vi "arm.vi"() -> ()   [LabVIEW 2014]
panel:
  in  "Controller Daisy Chain Position (1 - 4)":u8=1
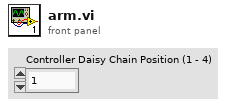
[diagram p1: front panel]
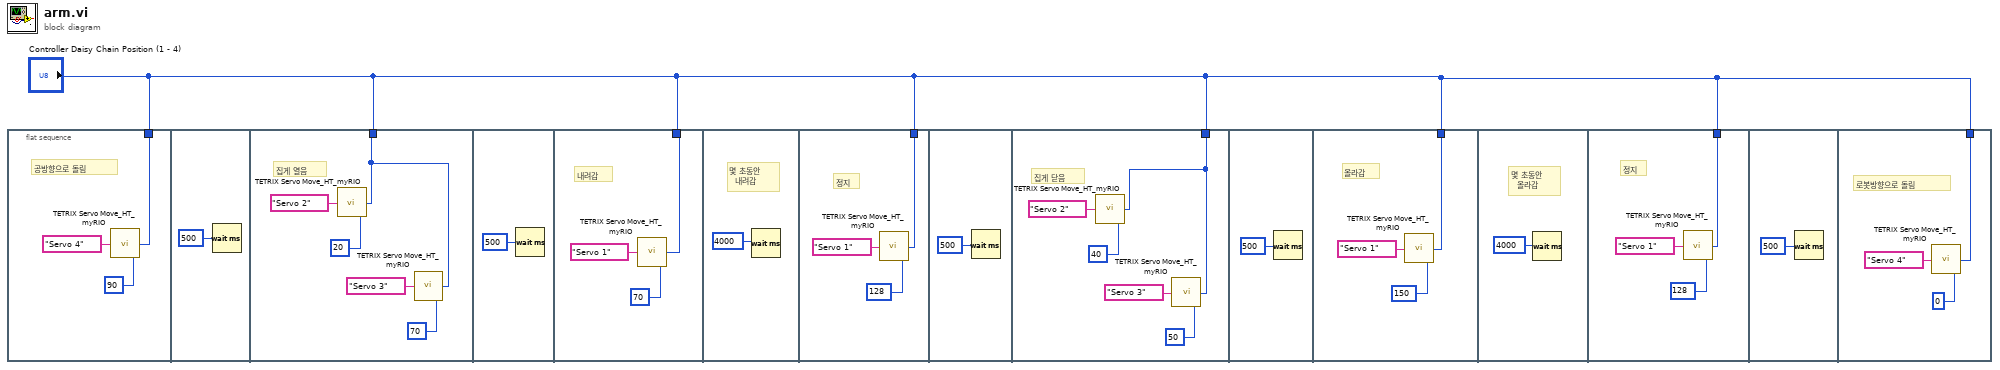
[diagram p0: block diagram]
diagram:
  n1 = flat-sequence {
    tunnel: "Controller Daisy Chain Position (1 - 4)" -> [w3]
    tunnel: "Controller Daisy Chain Position (1 - 4)" -> [w7]
    tunnel: "Controller Daisy Chain Position (1 - 4)" -> [w14]
    tunnel: "Controller Daisy Chain Position (1 - 4)" -> [w16]
    tunnel: "Controller Daisy Chain Position (1 - 4)" -> [w20]
    tunnel: "Controller Daisy Chain Position (1 - 4)" -> [w26]
    tunnel: "Controller Daisy Chain Position (1 - 4)" -> [w31]
    tunnel: "Controller Daisy Chain Position (1 - 4)" -> [w34]
    frame #0 {
      # "공방향으로 돌림"
      n2 = call <vilib>:"TETRIX Servo Move_HT_myRIO.vi"("Servo Position (0 - 255)"=u8 90, "Controller Daisy Chain Position (1 - 4)"=w3, "Select Servo"="Servo 4") -> ()  [unwired: 2 in, 1 out]
    }
    frame #1 {
      n3 = Wait (ms)(milliseconds to wait=u32 500 ("대기 시간(ms)")) -> ()  [unwired: 1 out]
    }
    frame #2 {
      # "집게 열음"
      n4 = call <vilib>:"TETRIX Servo Move_HT_myRIO.vi"("Servo Position (0 - 255)"=u8 20, "Controller Daisy Chain Position (1 - 4)"=w7, "Select Servo"="Servo 2") -> ()  [unwired: 2 in, 1 out]
      n5 = call <vilib>:"TETRIX Servo Move_HT_myRIO.vi"("Servo Position (0 - 255)"=u8 70, "Controller Daisy Chain Position (1 - 4)"=w7, "Select Servo"="Servo 3") -> ()  [unwired: 2 in, 1 out]
    }
    frame #3 {
      n6 = Wait (ms)(milliseconds to wait=u32 500 ("대기 시간(ms)")) -> ()  [unwired: 1 out]
    }
    frame #4 {
      # "내려감"
      n7 = call <vilib>:"TETRIX Servo Move_HT_myRIO.vi"("Servo Position (0 - 255)"=u8 70, "Controller Daisy Chain Position (1 - 4)"=w14, "Select Servo"="Servo 1") -> ()  [unwired: 2 in, 1 out]
    }
    frame #5 {
      # "몇 초동안\n  내려감"
      n8 = Wait (ms)(milliseconds to wait=u32 4000 ("대기 시간(ms)")) -> ()  [unwired: 1 out]
    }
    frame #6 {
      # "정지"
      n9 = call <vilib>:"TETRIX Servo Move_HT_myRIO.vi"("Servo Position (0 - 255)"=u8 128, "Controller Daisy Chain Position (1 - 4)"=w16, "Select Servo"="Servo 1") -> ()  [unwired: 2 in, 1 out]
    }
    frame #7 {
      n10 = Wait (ms)(milliseconds to wait=u32 500 ("대기 시간(ms)")) -> ()  [unwired: 1 out]
    }
    frame #8 {
      # "집게 닫음"
      n11 = call <vilib>:"TETRIX Servo Move_HT_myRIO.vi"("Servo Position (0 - 255)"=u8 40, "Controller Daisy Chain Position (1 - 4)"=w20, "Select Servo"="Servo 2") -> ()  [unwired: 2 in, 1 out]
      n12 = call <vilib>:"TETRIX Servo Move_HT_myRIO.vi"("Servo Position (0 - 255)"=u8 50, "Controller Daisy Chain Position (1 - 4)"=w20, "Select Servo"="Servo 3") -> ()  [unwired: 2 in, 1 out]
    }
    frame #9 {
      n13 = Wait (ms)(milliseconds to wait=u32 500 ("대기 시간(ms)")) -> ()  [unwired: 1 out]
    }
    frame #10 {
      # "올라감"
      n14 = call <vilib>:"TETRIX Servo Move_HT_myRIO.vi"("Servo Position (0 - 255)"=u8 150, "Controller Daisy Chain Position (1 - 4)"=w26, "Select Servo"="Servo 1") -> ()  [unwired: 2 in, 1 out]
    }
    frame #11 {
      # "몇 초동안\n  올라감"
      n15 = Wait (ms)(milliseconds to wait=u32 4000 ("대기 시간(ms)")) -> ()  [unwired: 1 out]
    }
    frame #12 {
      # "정지"
      n16 = call <vilib>:"TETRIX Servo Move_HT_myRIO.vi"("Servo Position (0 - 255)"=u8 128, "Controller Daisy Chain Position (1 - 4)"=w31, "Select Servo"="Servo 1") -> ()  [unwired: 2 in, 1 out]
    }
    frame #13 {
      n17 = Wait (ms)(milliseconds to wait=u32 500 ("대기 시간(ms)")) -> ()  [unwired: 1 out]
    }
    frame #14 {
      # "로봇방향으로 돌림"
      n18 = call <vilib>:"TETRIX Servo Move_HT_myRIO.vi"("Servo Position (0 - 255)"=u8 0, "Controller Daisy Chain Position (1 - 4)"=w34, "Select Servo"="Servo 4") -> ()  [unwired: 2 in, 1 out]
    }
  }
